vi "Get DMA FIFO from Target Name.vi"(5 "Expected Image Type":T1 items=["Grayscale (U8)", "Grayscale (I16)", "Grayscale (SGL)", "Complex (CSG)", "RGB (U32)", "HSL (U32)", "RGB (U64)", "Grayscale (U16)"], 6 "DMA FIFO Depth in Images":u32, 7 "DMA FIFO Name":string, 8 "error in (no error)":errorcluster, 9 "Image Size":T3, 10 "Image":T2, 11 "Refnum in":refnum<k20>) -> (0 "error out":errorcluster, 1 "DMA FIFO Size":u32, 2 "DMA FIFO from Target Name":string, 3 "Refnum out":refnum<k20>)   [LabVIEW 2017, in "NI_VDM_FPGA_Basics.lvlib"]
uses:
  <vilib>/visionFPGA/NI_VDM_FPGA_Basics.lvlib
  <vilib>/visionFPGA/Controls/IMAQ FPGA Image Size.ctl
  <vilib>/vision/Image Controls.llb/IMAQ Image.ctl
  <vilib>/NI/LVFPGA Adv Session Resources/LVFPGAAdvSessionResources.lvlib
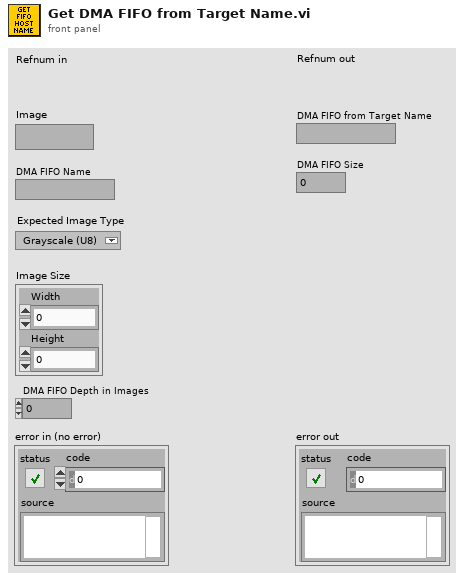
[diagram p1: front panel]
types:
  T1 = typedef "Image Type" = u32
  T2 = typedef "IMAQ Image.ctl" = refnum<image>
  T3 = typedef "IMAQ FPGA Image Size.ctl" = cluster{"Width":u32, "Height":u32}
  T4 = enum16{"Register", "Host To Target FIFO", "Target To Host FIFO"}
  T5 = typedef "LVFPGAAdvSessionResources.lvlib/ResourceInfo.ctl" = cluster{"Resource name":string, "Data type":variant, "Resource type":enum16{"Register", "Host To Target FIFO", "Target To Host FIFO"}}
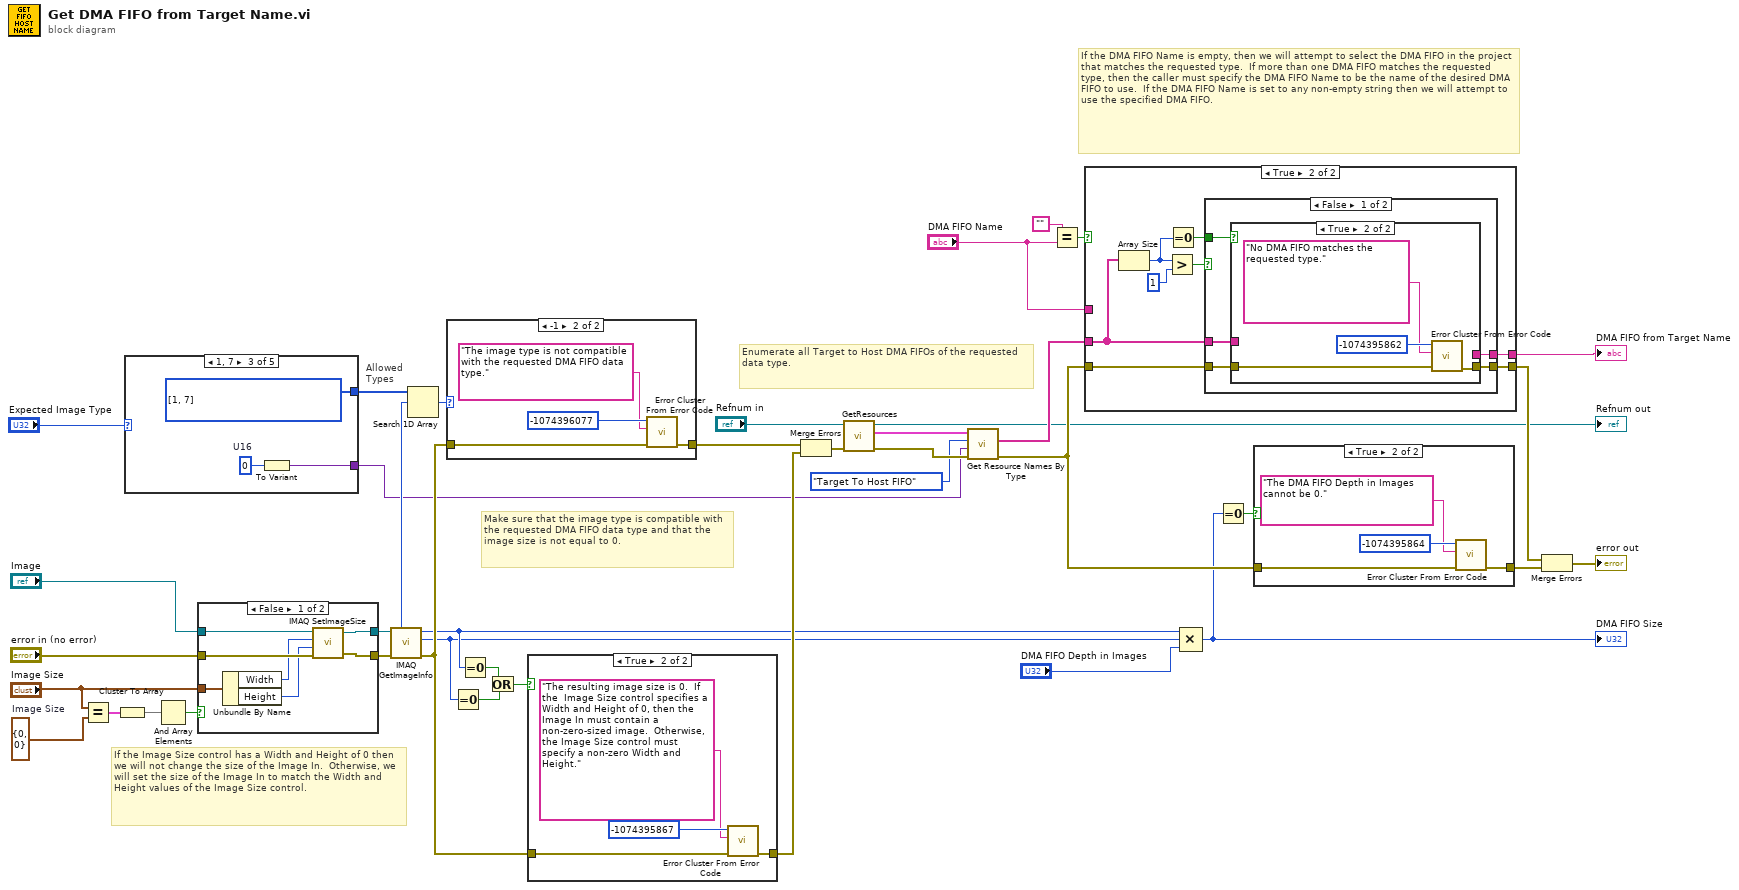
[diagram p0: block diagram]
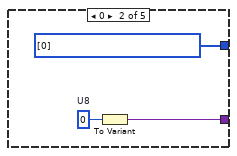
[diagram p3: hidden frame]
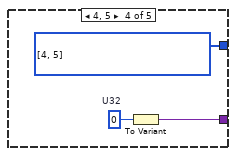
[diagram p4: hidden frame]
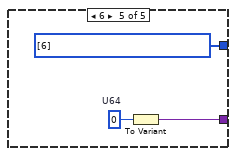
[diagram p5: hidden frame]
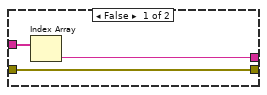
[diagram p11: hidden frame]
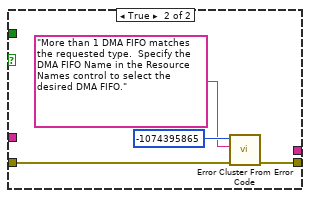
[diagram p12: hidden frame]
diagram:
  w21 = T3 {"Width"=0, "Height"=0}  # Image Size
  # "Allowed Types"
  # "Make sure that the image type is compatible with the requested DMA FIFO data type and that the image size is not equal to 0."
  # "If the Image Size control has a Width and Height of 0 then we will not change the size of the Image In.  Otherwise, we will set the size of the Image In to match the Width and Height values of the Image Size control."
  # "If the DMA FIFO Name is empty, then we will attempt to select the DMA FIFO in the project that matches the requested type.  If more than one DMA FIFO matches the requested type, then the caller must specify the DMA FIFO Name to be the name of the desired DMA FIFO to use.  If the DMA FIFO Name is set to any non-empty string then we will attempt to use the specified DMA FIFO."
  # "Enumerate all Target to Host DMA FIFOs of the requested data type."
  n1 = Equal?(x="Image Size", y=w21) -> (x = y?=w13:cluster{"Width":bool, "Height":bool})
  n2 = Cluster To Array(cluster=w13) -> (array=w14:bool[])
  n3 = case shown="1, 7" "Expected Image Type" {
    tunnel: [_ w42 w44 w47 w50] -> w1
    tunnel: [_ w41 w46 w49 w52] -> w3
    frame Default {
      # "Undefined type. Pass empty array of valid types."
    }
    frame 0 {
      w41 = T1[] [0] items=["Grayscale (U8)", "Grayscale (I16)", "Grayscale (SGL)", "Complex (CSG)", "RGB (U32)", "HSL (U32)", "RGB (U64)", "Grayscale (U16)"]
      w43 = u8 0  # U8
      n4 = To Variant(anything=w43) -> (Variant=w42:variant)
    }
    frame 1, 7 {
      w45 = u16 0  # U16
      w46 = T1[] [1, 7] items=["Grayscale (U8)", "Grayscale (I16)", "Grayscale (SGL)", "Complex (CSG)", "RGB (U32)", "HSL (U32)", "RGB (U64)", "Grayscale (U16)"]
      n5 = To Variant(anything=w45) -> (Variant=w44:variant)
    }
    frame 4, 5 {
      w48 = u32 0  # U32
      w49 = T1[] [4, 5] items=["Grayscale (U8)", "Grayscale (I16)", "Grayscale (SGL)", "Complex (CSG)", "RGB (U32)", "HSL (U32)", "RGB (U64)", "Grayscale (U16)"]
      n6 = To Variant(anything=w48) -> (Variant=w47:variant)
    }
    frame 6 {
      w51 = u64 0  # U64
      w52 = T1[] [6] items=["Grayscale (U8)", "Grayscale (I16)", "Grayscale (SGL)", "Complex (CSG)", "RGB (U32)", "HSL (U32)", "RGB (U64)", "Grayscale (U16)"]
      n7 = To Variant(anything=w51) -> (Variant=w50:variant)
    }
  }
  n8 = And Array Elements(Boolean array=w14) -> (logical AND=w15:bool)
  n9 = case shown="False" w15 {
    tunnel: "Image Size" -> [w57 _]
    tunnel: "Image" -> [w59 w61]
    tunnel: "error in (no error)" -> [w58 w60]
    tunnel: [w54 w61] -> w16
    tunnel: [w53 w60] -> w17
    frame False {
      n10 = Unbundle By Name(w57) -> ("Width"=w56:u32, "Height"=w55:u32)
      n11 = call "IMAQ SetImageSize"("error in (no error)"=w58, "Y Resolution"=w55, "X Resolution"=w56, "Image"=w59) -> ("error out"=w53:errorcluster, "Image Out"=w54:T2)  [unwired: 1 in]
    }
    frame True {
    }
  }
  n12 = call "IMAQ GetImageInfo"("error in (no error)"=w17, "Image"=w16) -> ("error out"=w27:errorcluster, "Y Resolution"=w25:i32, "X Resolution"=w26:i32, "Image Type"=w4:T1)  [unwired: 2 in, 4 out]
  n13 = Search 1D Array(1D array=w3, element=w4) -> (index of element=w2:i32)  [unwired: 1 in]
  n14 = case shown="-1" w2 {
    tunnel: w27 -> [w62 w64]
    tunnel: [w62 w63] -> w29
    frame Default {
    }
    frame -1 {
      n15 = call <vilib>:"Error Cluster From Error Code.vi"("error in (no error)"=w64, "error message (\"\")"="The image type is not compatible with the requested DMA FIFO data type." ("error message (\"\")"), "error code (0)"=-1074396077) -> ("error out"=w63:errorcluster)  [unwired: 6 in]
    }
  }
  n16 = Equal To 0?(x=w25) -> (x = 0?=w23:bool)
  n17 = Equal To 0?(x=w26) -> (x = 0?=w22:bool)
  n18 = Or(x=w22, y=w23) -> (x .or. y?=w24:bool)
  n19 = case shown="True" w24 {
    tunnel: w27 -> [w67 w69]
    tunnel: [w67 w68] -> w30
    frame False {
    }
    frame True {
      n20 = call <vilib>:"Error Cluster From Error Code.vi"("error in (no error)"=w69, "error message (\"\")"="The resulting image size is 0.  If the  Image Size control specifies a Width and Height of 0, then the Image In must contain a non-zero-sized image.  Otherwise, the Image Size control must specify a non-zero Width and Height." ("error message (\"\")"), "error code (0)"=-1074395867) -> ("error out"=w68:errorcluster)  [unwired: 6 in]
    }
  }
  n21 = Merge Errors(w29, w30) -> (w28:errorcluster)
  n22 = call <vilib>:"GetResources.vi"("error in (no error)"=w28, "FPGA VI Reference in"="Refnum in") -> ("error out"=w38:errorcluster, "Resource info out"=w37:T5[], "FPGA VI Reference out"=→"Refnum out":refnum<k20>)  [unwired: 7 in]
  n23 = call <vilib>:"Get Resource Names By Type.vi"("error in (no error)"=w38, "Data Type"=w1, "Resource Type"=T4."Target To Host FIFO", "Resource Info In"=w37) -> ("error out"=w40:errorcluster, "Resource Names"=w39:string[])  [unwired: 5 in, 1 out]
  n24 = Equal?(x="", y="DMA FIFO Name") -> (x = y?=w7:bool)
  n25 = case shown="True" w7 {
    tunnel: w39 -> [_ w76]
    tunnel: w40 -> [w72 w79]
    tunnel: [w72 w80] -> w34
    tunnel: [w73 w78] -> w8
    tunnel: "DMA FIFO Name" -> [w73 _]
    frame False {
    }
    frame True {
      n26 = Array Size(array=w76) -> (size(s)=w74:i32)
      n27 = Greater?(x=w74, y=1 ("x")) -> (0:w77:bool)
      n28 = Equal To 0?(x=w74) -> (x = 0?=w75:bool)
      n29 = case shown="False" w77 {
        tunnel: w76 -> [w86 _]
        tunnel: [w85 _] -> w78
        tunnel: [w83 w95] -> w80
        tunnel: w79 -> [w84 w94]
        tunnel: w75 -> [w82 _]
        frame False {
          n30 = case shown="True" w82 {
            tunnel: w86 -> [w89 _]
            tunnel: [w88 _] -> w85
            tunnel: w84 -> [w87 w90]
            tunnel: [w87 w91] -> w83
            frame False {
              n31 = Index Array(array=w89) -> (element=w88:string)  [unwired: 1 in]
            }
            frame True {
              n32 = call <vilib>:"Error Cluster From Error Code.vi"("error in (no error)"=w90, "error message (\"\")"="No DMA FIFO matches the requested type." ("error message (\"\")"), "error code (0)"=-1074395862) -> ("error out"=w91:errorcluster)  [unwired: 6 in]
            }
          }
        }
        frame True {
          n33 = call <vilib>:"Error Cluster From Error Code.vi"("error in (no error)"=w94, "error message (\"\")"="More than 1 DMA FIFO matches the requested type.  Specify the DMA FIFO Name in the Resource Names control to select the desired DMA FIFO." ("error message (\"\")"), "error code (0)"=-1074395865) -> ("error out"=w95:errorcluster)  [unwired: 6 in]
        }
      }
    }
  }
  "DMA FIFO from Target Name" <- w8
  n34 = Compound Arithmetic op=MULTIPLY(w26, w25, "DMA FIFO Depth in Images") -> (w32:u32)
  "DMA FIFO Size" <- w32
  n35 = Equal To 0?(x=w32) -> (x = 0?=w31:bool)
  n36 = case shown="True" w31 {
    tunnel: [w98 w100] -> w35
    tunnel: w40 -> [w98 w99]
    frame False {
    }
    frame True {
      n37 = call <vilib>:"Error Cluster From Error Code.vi"("error in (no error)"=w99, "error message (\"\")"="The DMA FIFO Depth in Images cannot be 0." ("error message (\"\")"), "error code (0)"=-1074395864) -> ("error out"=w100:errorcluster)  [unwired: 6 in]
    }
  }
  n38 = Merge Errors(w34, w35) -> (→"error out":errorcluster)
